vi "Execute.vi"(8 "error in (no error)":errorcluster, 10 "System In":refnum<class "abs_System.lvclass">, 11 "Node in":refnum<class "Test Log.lvclass">) -> (0 "error out":errorcluster, 1 "Status":T1, 2 "System Out":refnum<class "abs_System.lvclass">, 3 "Node out":refnum<class "Test Log.lvclass">)   [LabVIEW 2021, in "Test Log.lvclass"]
uses:
  Test Log.lvclass
  C:/Users/Tim/Documents/LabVIEW/2021/Behaviour Tree/Source/abs_Log/abs_Log.lvclass
  abs_Node/Status.ctl
  abs_System/abs_System.lvclass
  Test System/Test System.lvclass
  C:/Users/Tim/Documents/LabVIEW/2021/Behaviour Tree/Source/abs_System/abs_System.lvclass
  abs_Log/abs_Log.lvclass/abs_Log.ctl
  Test System/Test System.lvclass/Test System.ctl
  abs_Log/Properties/Read Message.vi
  Test System/Properties/Read Log Messages.vi
  Test System/Properties/Write Log Messages.vi
  abs_Node/abs_Node.lvclass
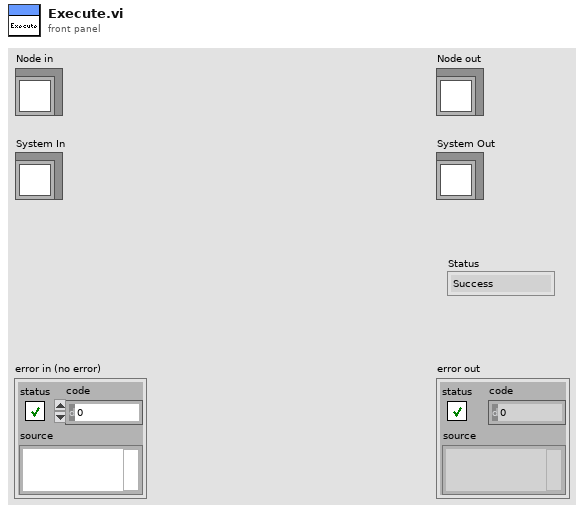
[diagram p1: front panel]
types:
  T1 = typedef "BT.lvlib/abs_Node.lvclass/Status.ctl" = enum16{"Success", "Failure", "Running"}
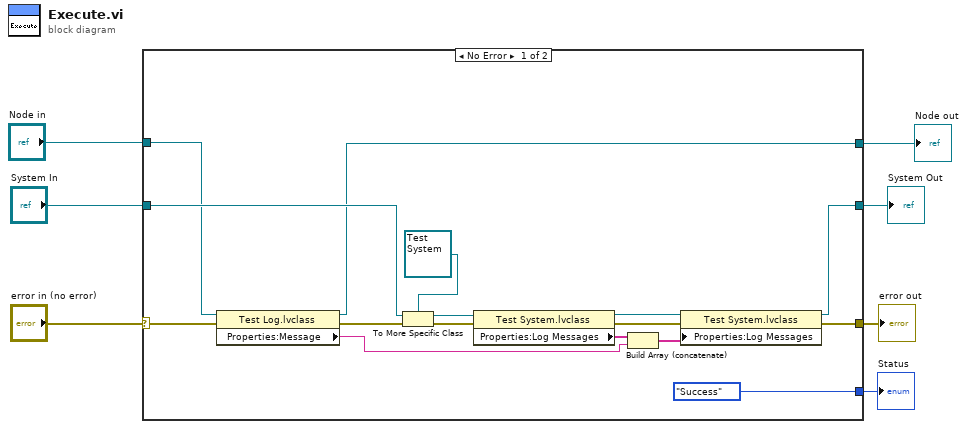
[diagram p0: block diagram]
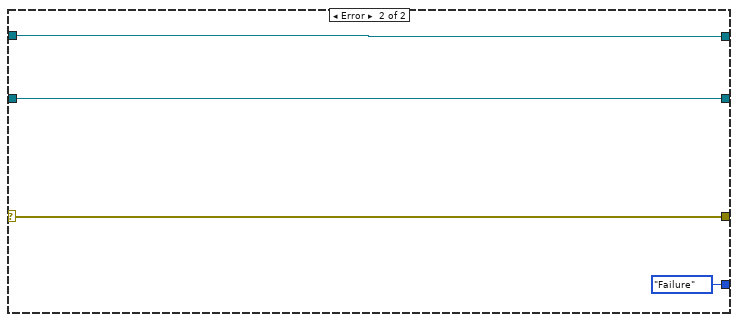
[diagram p2: hidden frame]
diagram:
  n1 = case shown="No Error" "error in (no error)" {
    selector: "error in (no error)" -> [w18 w25]
    tunnel: "System In" -> [w23 w26]
    tunnel: "Node in" -> [w17 w27]
    tunnel: [w16 w27] -> w4
    tunnel: [w10 w25] -> w3
    tunnel: [Status."Success" ("Status") Status."Failure" ("Status")] -> w2
    tunnel: [w8 w26] -> w1
    frame No Error {
      n2 = property class="Test Log.lvclass"(reference=w17, error in=w18) -> (reference out=w16:refnum<class "Test Log.lvclass">, error out=w19:errorcluster, "Properties:Message"=w11:string)
      n3 = To More Specific Class(target class=refnum<class "Test System.lvclass"> refnum ("Test System.lvclass"), reference=w23, error in=w19) -> (specific class reference=w20:refnum<class "Test System.lvclass">, error out=w21:errorcluster)
      n4 = property class="Test System.lvclass"(reference=w20, error in=w21) -> (reference out=w15:refnum<class "Test System.lvclass">, error out=w14:errorcluster, "Properties:Log Messages"=w13:string[])
      n5 = Build Array (concatenate)(w13, w11) -> (w12:string[])
      n6 = property class="Test System.lvclass"(reference=w15, error in=w14, "Properties:Log Messages"=w12) -> (reference out=w8:refnum<class "Test System.lvclass">, error out=w10:errorcluster)
    }
    frame Error {
    }
  }
  "error out" <- w3
  "Node out" <- w4
  "Status" <- w2
  "System Out" <- w1
